vi "Create Room Service Request.vi"(0 "Room Service Manager Model in":refnum<class "Room Service Manager Model.lvclass">, 5 "Room Service":refnum<class "Room Service Base.lvclass">, 11 "error in (no error)":errorcluster) -> (4 "Room Service Manager Model out":refnum<class "Room Service Manager Model.lvclass">, 15 "error out":errorcluster)   [LabVIEW 2023, in "Room Service Manager Model.lvlib" / "Room Service Manager Model.lvclass"]
uses:
  Room Service Manager Model.lvclass
  Room Service Manager Model.lvclass/Room Service Manager Model.ctl
  Interfaces/Incoming Hotel Management Tool Model Interface Messages/Create Room Service Request Msg/Create Room Service Request Msg.lvclass
  <vilib>/ActorFramework/Actor/Actor.lvclass
  C:/Users/bhaghyaraj/Trainings/NI Actor Framework/SDLC/Model Base/Model Base/Model Base.lvclass
  C:/Program Files/National Instruments/LabVIEW 2023/vi.lib/ActorFramework/Actor/Actor.lvclass
  C:/Users/bhaghyaraj/Trainings/NI Actor Framework/SDLC/Interfaces/Model Base/Incoming Model Base Interface.lvclass
  C:/Users/bhaghyaraj/Trainings/NI Actor Framework/SDLC/Room Service Manager Model/Room Service Manager Model/Room Service Manager Model.lvclass
  Room Service Types/Room Service Base/Room Service Base.lvclass
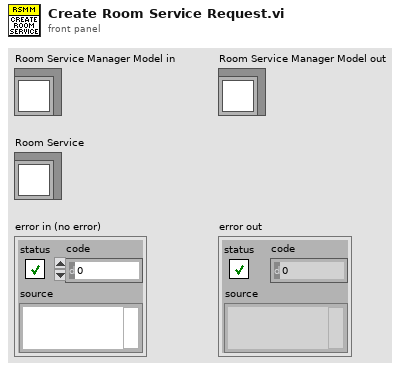
[diagram p1: front panel]
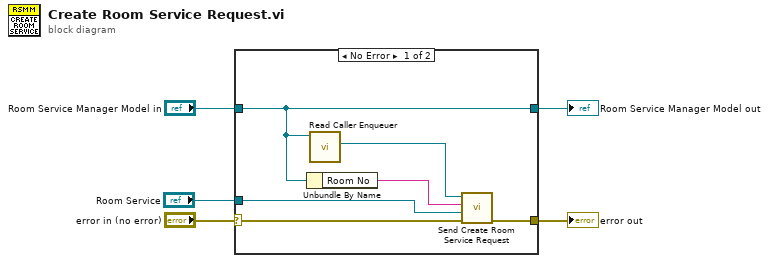
[diagram p0: block diagram]
diagram:
  n1 = case shown="No Error" "error in (no error)" {
    selector: "error in (no error)" -> [w11 w13]
    tunnel: [w10 w13] -> w2
    tunnel: [w8 w12] -> w3
    tunnel: "Room Service Manager Model in" -> [w8 w12]
    tunnel: "Room Service" -> [w6 _]
    frame No Error {
      n2 = Unbundle By Name(w8) -> ("Room No"=w7:string)
      n3 = call <vilib>:"Read Caller Enqueuer.vi"("Actor"=w8) -> ("Caller Enqueuer"=w9:refnum<class "Message Enqueuer.lvclass">)  [unwired: 10 in]
      n4 = call "Send Create Room Service Request.vi"("error in (no error)"=w11, "Room Service"=w6, "Rooms No"=w7, "Message Enqueuer"=w9) -> ("error out"=w10:errorcluster)  [unwired: 6 in, 1 out]
    }
    frame Error {
    }
  }
  "error out" <- w2
  "Room Service Manager Model out" <- w3
